vi "NaNCorrect.vi"(8 "error in (no error)":errorcluster, 9 "Value":dbl=10.0 format="%#_13g", 10 "CorrectAll":bool, 11 "Control-Client in":refnum<class "Control-Client.lvclass">) -> (0 "error out":errorcluster, 3 "Control-Client out":refnum<class "Control-Client.lvclass">)   [LabVIEW 2015, in "Control-Client.lvclass"]
uses:
  Control-Client.lvclass
  Control-Client.lvclass/Control-Client.ctl
  methods/Read Group #.vi
  Experiments/Experiments_group.lvclass
  Experiments/Experiment.lvclass
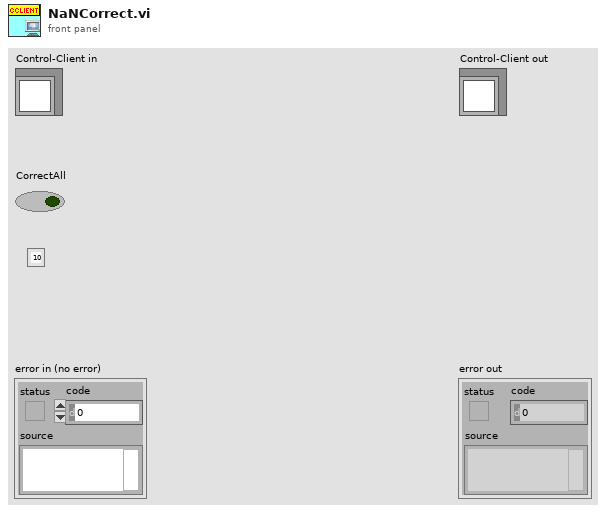
[diagram p1: front panel]
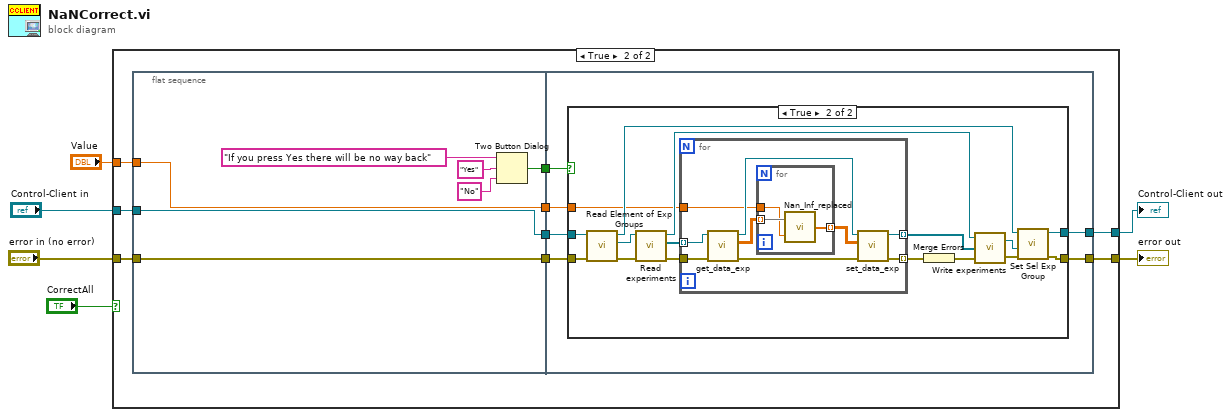
[diagram p0: block diagram]
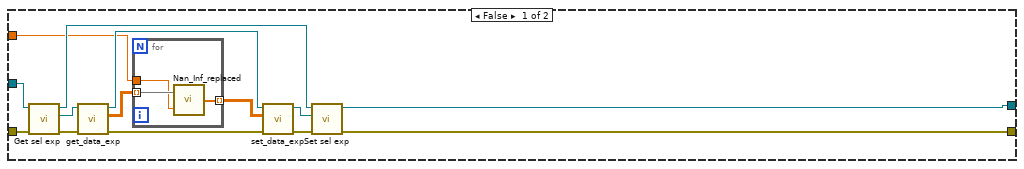
[diagram p2: hidden frame]
diagram:
  n1 = case shown="True" "CorrectAll" {
    tunnel: "Control-Client in" -> [w14 w29]
    tunnel: [w13 w31] -> w5
    tunnel: [w12 w32] -> w4
    tunnel: "error in (no error)" -> [w8 w28]
    tunnel: "Value" -> [w7 w30]
    frame False {
      n2 = call "Get sel exp.vi"("error in (no error)"=w8, "Control-Client in"=w14) -> ("error out"=w9:errorcluster, "Sel experiment"=w19:refnum<class "Experiment.lvclass">, "Control-Client out"=w16:refnum<class "Control-Client.lvclass">)  [unwired: 7 in]
      n3 = call "get_data_exp.vi"("error in (no error)"=w9, "Experiment.lvclass in"=w19) -> ("error out"=w10:errorcluster, "Data"=w18:sgl[][], "Experiment.lvclass out"=w15:refnum<class "Experiment.lvclass">)  [unwired: 7 in]
      n4 = for {
        tunnel: w18 -> [w23] mode=indexing
        tunnel: [w22] -> w17 mode=indexing
        tunnel: w7 -> [w21]
        n5 = call "Nan_Inf_replaced.vi"("Value"=w21, "IN with Inf and NaN"=w23) -> ("Out with NaN and Inf replaced"=w22:dbl[])
      }
      n6 = call "set_data_exp.vi"("error in (no error)"=w10, "Data"=w17, "Experiment.lvclass in"=w15) -> ("error out"=w11:errorcluster, "Experiment.lvclass out"=w20:refnum<class "Experiment.lvclass">)  [unwired: 7 in]
      n7 = call "Set sel exp.vi"("error in (no error)"=w11, "Experiment"=w20, "Control-Client in"=w16) -> ("error out"=w12:errorcluster, "Control-Client out"=w13:refnum<class "Control-Client.lvclass">)  [unwired: 7 in]
    }
    frame True {
      n8 = flat-sequence {
        tunnel: w28 -> [w37]
        tunnel: w29 -> [w38]
        tunnel: w30 -> [w39]
        tunnel: [w39] -> w27
        tunnel: [w38] -> w26
        tunnel: [w37] -> w25
        tunnel: [w33] -> w24
        tunnel: [w45] -> w32
        tunnel: [w44] -> w31
        tunnel: w27 -> [w43]
        tunnel: w26 -> [w42]
        tunnel: w25 -> [w41]
        tunnel: w24 -> [w40]
        frame #0 {
          n9 = Two Button Dialog(message="If you press Yes there will be no way back", 1:"No" ("F button name (\"Cancel\")"), 2:"Yes" ("T button name (\"OK\")")) -> (T button?=w33:bool)
        }
        frame #1 {
          n10 = case shown="True" w40 {
            tunnel: [w46 w52] -> w45
            tunnel: [w47 w51] -> w44
            tunnel: w43 -> [_ w50]
            tunnel: w42 -> [w47 w49]
            tunnel: w41 -> [w46 w48]
            frame False {
            }
            frame True {
              n11 = call "Read Element of Exp Groups.vi"("error in (no error)"=w48, "Control-Client in"=w49) -> ("error out"=w54:errorcluster, "Experiments_group.lvclass"=w53:refnum<class "Experiments_group.lvclass">, "Control-Client out"=w62:refnum<class "Control-Client.lvclass">)  [unwired: 7 in]
              n12 = call "Read experiments.vi"("error in (no error)"=w54, "Experiments_group.lvclass in"=w53) -> ("error out"=w55:errorcluster, "Experiments"=w56:refnum<class "Experiment.lvclass">[], "Experiments_group.lvclass out"=w57:refnum<class "Experiments_group.lvclass">)  [unwired: 6 in]
              n13 = for {
                tunnel: w55 -> [w65]
                tunnel: w56 -> [w66] mode=indexing
                tunnel: [w67] -> w58 mode=indexing
                tunnel: [w68] -> w59 mode=indexing
                tunnel: w50 -> [w64]
                n14 = call "get_data_exp.vi"("error in (no error)"=w65, "Experiment.lvclass in"=w66) -> ("error out"=w69:errorcluster, "Data"=w72:sgl[][], "Experiment.lvclass out"=w70:refnum<class "Experiment.lvclass">)  [unwired: 7 in]
                n15 = for {
                  tunnel: w72 -> [w75] mode=indexing
                  tunnel: [w74] -> w71 mode=indexing
                  tunnel: w64 -> [w73]
                  n16 = call "Nan_Inf_replaced.vi"("Value"=w73, "IN with Inf and NaN"=w75) -> ("Out with NaN and Inf replaced"=w74:dbl[])
                }
                n17 = call "set_data_exp.vi"("error in (no error)"=w69, "Data"=w71, "Experiment.lvclass in"=w70) -> ("error out"=w68:errorcluster, "Experiment.lvclass out"=w67:refnum<class "Experiment.lvclass">)  [unwired: 7 in]
              }
              n18 = Merge Errors(w59) -> (w60:errorcluster)
              n19 = call-dynamic "Write experiments.vi"("error in (no error)"=w60, "Experiments"=w58, "Experiments_group.lvclass in"=w57) -> ("error out"=w63:errorcluster, "Experiments_group.lvclass out"=w61:refnum<class "Experiments_group.lvclass">)
              n20 = call "Set Sel Exp Group.vi"("error in (no error)"=w63, "Exp Group"=w61, "Control-Client in"=w62) -> ("error out"=w52:errorcluster, "Control-Client out"=w51:refnum<class "Control-Client.lvclass">)  [unwired: 7 in]
            }
          }
        }
      }
    }
  }
  "error out" <- w4
  "Control-Client out" <- w5
